vi "extract From Input Packet ENC Pos.vi"(10 "channel":i32, 11 "instance":i32) -> (3 "function return":i32)   [LabVIEW 2025, in "SADI_FW3.lvlib"]
doc: "SADI_API_Wrapper uint32_t extractFromInputPacket_ENCPos(int instance,int channel);\nSADI_API_Wrapper int32_t extractFromInputPacket_ENCPos(int instance,int channel);"
uses:
  SADI_FW3.lvlib
  SADI_FW3.dll
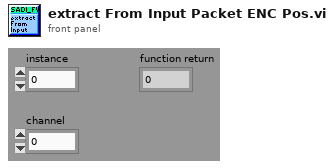
[diagram p1: front panel]
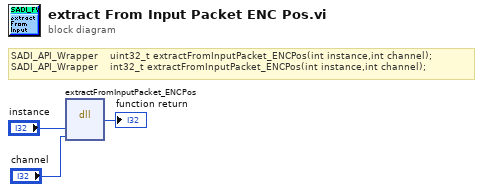
[diagram p0: block diagram]
diagram:
  # "SADI_API_Wrapper    uint32_t extractFromInputPacket_ENCPos(int instance,int channel);\nSADI_API_Wrapper    int32_t extractFromInputPacket_ENCPos(int instance,int channel);"
  n1 = dll-call lib="C:/Users/noaht/School/Fall 2025/Controls Lab/Lab 3/EML4314c_FA25_framework_0/LVLib/SADI_FW3.*" fn="extractFromInputPacket_ENCPos"("instance"="instance", "channel"="channel") -> ("return type"=→"function return":i32)  [unwired: 5 in, 2 out]
